vi "Open-Close.vi"(4 "Remote Path":string, 5 "Username":string, 6 "Password":string, 7 "Address":string, 8 "Error In":errorcluster) -> (0 "Error Out":errorcluster)   [LabVIEW 2018, in "Tests.lvlib" / "SFTP Directory.lvlib"]
uses:
  SFTP Directory.lvlib
  <vilib>/addons/_JKI Toolkits/Caraya/classes/Test/Test.lvclass
  <vilib>/addons/_JKI Toolkits/Caraya/classes/Assert/Assert.lvclass
  Tests.lvlib
  src/Toolkit/API/SFTP Directory/SFTP Directory.lvclass
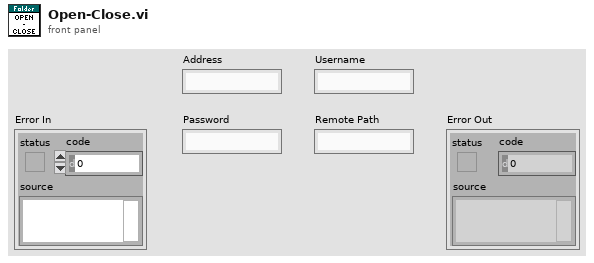
[diagram p1: front panel]
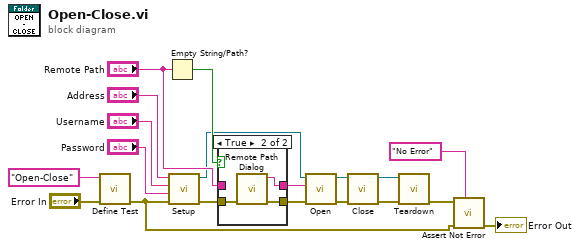
[diagram p0: block diagram]
diagram:
  n1 = call <vilib>:"Define Test.vi"("error in (no error)"="Error In", "Label (VI Title)"="Open-Close") -> ("error out"=w13:errorcluster)  [unwired: 9 in]
  n2 = Empty String/Path?(string/path="Remote Path") -> (empty?=w15:bool)
  n3 = call "Setup.vi"("Error In"=w13, "Password"="Password", "Username"="Username", "Address"="Address") -> ("Error Out"=w12:errorcluster, "SFTP"=w2:refnum<class "SFTP.lvclass">)  [unwired: 6 in]
  n4 = case shown="True" w15 {
    tunnel: [w20 w24] -> w10
    tunnel: [w21 w23] -> w11
    tunnel: "Remote Path" -> [w21 _]
    tunnel: w12 -> [w20 w22]
    frame False {
    }
    frame True {
      n5 = call "Remote Path Dialog.vi"("Error In"=w22) -> ("Error Out"=w24:errorcluster, "Remote Path Out"=w23:string)  [unwired: 9 in]
    }
  }
  n6 = call "Open.vi"("Error In"=w10, "Remote Path"=w11, "SFTP"=w2) -> ("Error Out"=w9:errorcluster, "SFTP Directory"=w8:refnum<class "SFTP Directory.lvclass">)  [unwired: 7 in]
  n7 = call "Close.vi"("Error In"=w9, "SFTP Directory"=w8) -> ("Error Out"=w7:errorcluster, "SFTP"=w1:refnum<class "SFTP.lvclass">)  [unwired: 8 in]
  n8 = call "Teardown.vi"("Error In"=w7, "SFTP"=w1) -> ("Error Out"=w6:errorcluster)  [unwired: 9 in]
  n9 = call <vilib>:"Assert Not Error.vi"("Label"="No Error", "error in (no error)"=w13, "Not Error?"=w6) -> ("error out"=→"Error Out":errorcluster)  [unwired: 8 in]
